vi "GlobalConAxisPI.vi"() -> ()   [LabVIEW 2013]
panel:
  out "Conn. Axes":string[](array[string])
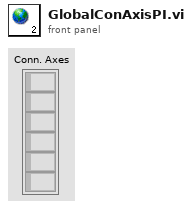
[diagram p1: front panel]
diagram:
